vi "blePIP.vi"   [LabVIEW 2018]
uses:
  Global_1259.vi
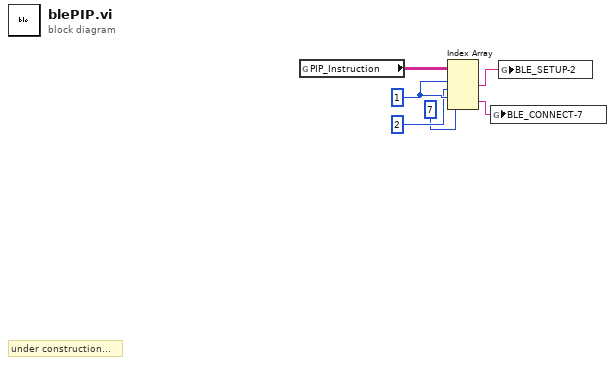
[diagram p0: block diagram]
diagram:
  w3 = 1 ("index (row)")
  # "under construction..."
  n1 = global read "Global_1259.vi" "PIP_Instruction"() -> (w6:string[][])
  n2 = Index Array(array=w6, index (row) #1=w3, index (col) #1=2 ("disabled index (col)"), index (row) #2=w3, index (col) #2=7 ("disabled index (col)")) -> (element #1=w5:string, element #2=w4:string)
  n3 = global write "Global_1259.vi" "BLE_CONNECT-7"(w4) -> ()
  n4 = global write "Global_1259.vi" "BLE_SETUP-2"(w5) -> ()
